vi "CRYCalc maximum.vi"(6 "Work in":u16, 7 "Step Setup VI No":i32, 8 "Statistic Run Number":i32, 11 "Data in":T1 {"Z data" items=["dB", "Lin"]; "X data" items=["dB", "Lin"]; "Y data" items=["dB", "Lin"]; "Z dB ref" format="%.1f"; "Z axis" items=["Log", "Lin"]; "X dB ref" format="%.1f"; "X axis" items=["Log", "Lin"]; "Y axis" items=["Log", "Lin"]; "Y dB ref" format="%.1f"; "Curve"."z" format="%.2f"; "Curve"."y" format="%.2f"; "Curve"."x" format="%.2f"}) -> (3 "Maximum Out":T1 {"Z data" items=["dB", "Lin"]; "X data" items=["dB", "Lin"]; "Y data" items=["dB", "Lin"]; "Z dB ref" format="%.1f"; "Z axis" items=["Log", "Lin"]; "X dB ref" format="%.1f"; "X axis" items=["Log", "Lin"]; "Y axis" items=["Log", "Lin"]; "Y dB ref" format="%.1f"; "Curve"."z" format="%.2f"; "Curve"."y" format="%.2f"; "Curve"."x" format="%.2f"})   [LabVIEW 2013]
uses:
  Typedef Control/CRYData Cluster Array.ctl
  Typedef Control/CRYData Cluster.ctl
  CRYStatistics Global.vi
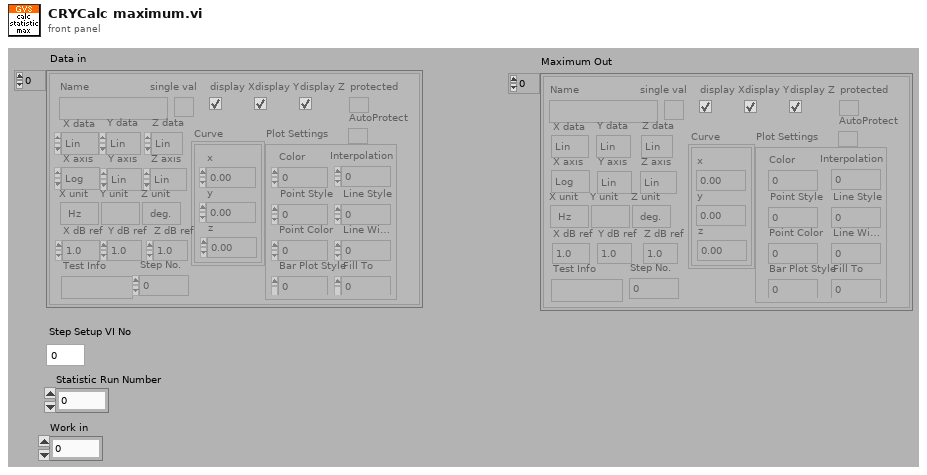
[diagram p1: front panel]
types:
  T1 = typedef "CRYData Cluster Array.ctl" = T2[]
  T2 = typedef "CRYData Cluster.ctl" = cluster{"Name":string, "Curve":cluster{"x":dbl, "y":dbl, "z":dbl}[], "X data":u16, "Y data":u16, "Z data":u16, "X axis":u16, "Y axis":u16, "Z axis":u16, "X unit":string, "Y unit":string, "Z unit":string, "X dB ref":dbl, "Y dB ref":dbl, "Z dB ref":dbl, "single val":bool, "protected":bool, "display X":bool, "display Y":bool, "display Z":bool, "Test Info":string, "Step No.":i32, "Plot Settings":cluster{"Color":u32, "Interpolation":u8, "Point Style":u8, "Line Style":u8, "Point Color":u32, "Line Width":u8, "Bar Plot Style":u8, "Fill To":i16}, "AutoProtect":bool}
  T3 = enum32{"English", "Chinese", "Korean", "Japanese", "Russian", "Chinese traditional"}
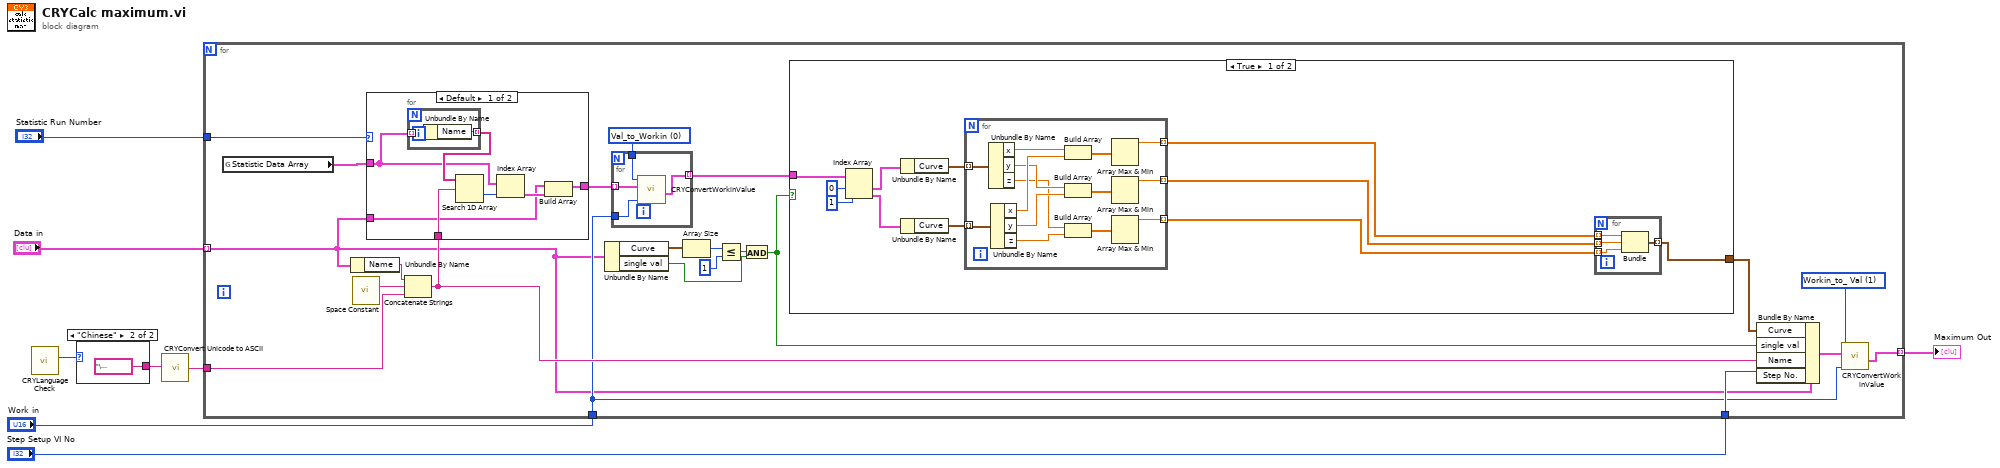
[diagram p0: block diagram]
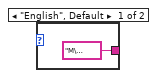
[diagram p2: hidden frame]
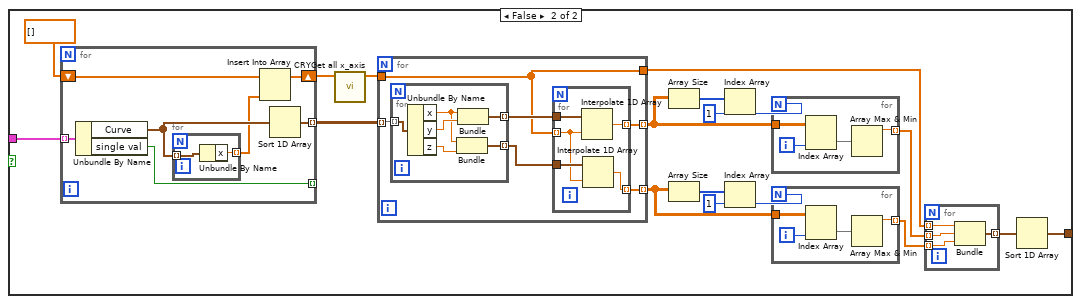
[diagram p3: hidden frame]
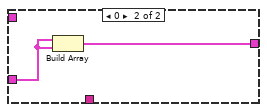
[diagram p4: hidden frame]
diagram:
  n1 = call "CRYLanguage Check.vi"() -> ("Language"=w4:T3)  [unwired: 10 in, 1 out]
  n2 = case shown="\"Chinese\"" w4 {
    tunnel: ["M\u0000a\u0000x\u0000" ("format string") "\u0000g'Y<P" ("format string")] -> w5
    frame "English", Default {
    }
    frame "Chinese" {
    }
  }
  n3 = call "CRYConvert Unicode to ASCII.vi"("Unicode"=w5) -> ("ASCII"=w3:string)  [unwired: 4 in]
  n4 = for {
    tunnel: "Data in" -> [w12] mode=indexing
    tunnel: [w21] -> w1 mode=indexing
    tunnel: "Step Setup VI No" -> [w30]
    tunnel: "Statistic Run Number" -> [w29]
    tunnel: w3 -> [w28]
    tunnel: "Work in" -> [w20]
    w18 = u16 1 items=["Val_to_Workin", "Workin_to_ Val"] ("Type")
    w19 = u16 0 items=["Val_to_Workin", "Workin_to_ Val"] ("Type")
    n5 = global read "CRYStatistics Global.vi" "Statistic Data Array"() -> (w25:T1)
    n6 = Unbundle By Name(w12) -> ("Name"=w26:string)
    n7 = call <vilib>:"Space Constant.vi"() -> ("String"=w27:string)
    n8 = Concatenate Strings(w26, w27, w28) -> (w31:string)
    n9 = case shown="Default" w29 {
      tunnel: w12 -> [w123 w132]
      tunnel: [w125 w131] -> w24
      tunnel: w31 -> [w128 _]
      tunnel: w25 -> [w122 _]
      frame Default {
        n10 = for {
          tunnel: w122 -> [w130] mode=indexing
          tunnel: [w129] -> w127 mode=indexing
          n11 = Unbundle By Name(w130) -> ("Name"=w129:string)
        }
        n12 = Search 1D Array(1D array=w127, element=w128) -> (index of element=w126:i32)  [unwired: 1 in]
        n13 = Index Array(array=w122, index=w126) -> (element=w124:T2)
        n14 = Build Array(w123, w124) -> (w125:T2[])
      }
      frame 0 {
        n15 = Build Array(w132, w132) -> (w131:T2[])
      }
    }
    n16 = Unbundle By Name(w12) -> ("Curve"=w13:cluster{"x":dbl, "y":dbl, "z":dbl}[], "single val"=w17:bool)
    n17 = for {
      tunnel: w24 -> [w121] mode=indexing
      tunnel: [w120] -> w23 mode=indexing
      tunnel: w19 -> [w119]
      tunnel: w20 -> [w118]
      n18 = call "CRYConvertWorkinValue.vi"("Work in"=w118, "In"=w121, "Type"=w119) -> ("Out"=w120:T2)  [unwired: 8 in]
    }
    n19 = Array Size(array=w13) -> (size(s)=w14:i32)
    n20 = Less Or Equal?(x=w14, y=1) -> (x <= y?=w16:bool)
    n21 = And(x=w16, y=w17) -> (x .and. y?=w11:bool)
    n22 = case shown="True" w11 {
      tunnel: [w33 w69] -> w32
      tunnel: w23 -> [w43 w62]
      frame True {
        n23 = Index Array(array=w43, index #1=0 ("index"), index #2=1 ("index")) -> (element #1=w40:T2, element #2=w39:T2)
        n24 = Unbundle By Name(w40) -> ("Curve"=w38:cluster{"x":dbl, "y":dbl, "z":dbl}[])
        n25 = Unbundle By Name(w39) -> ("Curve"=w37:cluster{"x":dbl, "y":dbl, "z":dbl}[])
        n26 = for {
          tunnel: w38 -> [w57] mode=indexing
          tunnel: w37 -> [w56] mode=indexing
          tunnel: [w46] -> w36 mode=indexing
          tunnel: [w45] -> w35 mode=indexing
          tunnel: [w44] -> w34 mode=indexing
          n27 = Unbundle By Name(w57) -> ("x"=w55:dbl, "y"=w53:dbl, "z"=w51:dbl)
          n28 = Unbundle By Name(w56) -> ("x"=w54:dbl, "y"=w52:dbl, "z"=w50:dbl)
          n29 = Build Array(w55, w54) -> (w49:dbl[])
          n30 = Build Array(w53, w52) -> (w48:dbl[])
          n31 = Build Array(w51, w50) -> (w47:dbl[])
          n32 = Array Max & Min(array=w49) -> (max value=w46:dbl)  [unwired: 3 out]
          n33 = Array Max & Min(array=w48) -> (max value=w45:dbl)  [unwired: 3 out]
          n34 = Array Max & Min(array=w47) -> (max value=w44:dbl)  [unwired: 3 out]
        }
        n35 = for {
          tunnel: [w61] -> w33 mode=indexing
          tunnel: w36 -> [w60] mode=indexing
          tunnel: w35 -> [w59] mode=indexing
          tunnel: w34 -> [w58] mode=indexing
          n36 = Bundle(w60, w59, w58) -> (w61:cluster{dbl, dbl, dbl})  [unwired: 1 out]
        }
      }
      frame False {
        n37 = for {
          tunnel: [w92] -> w76 mode=indexing
          tunnel: w62 -> [w93] mode=indexing
          shift-right: [w96] -> w68
          shift-left: dbl[] [] ("x_Array") -> [w95]
          tunnel: [w94] -> _ mode=indexing
          n38 = Unbundle By Name(w93) -> ("Curve"=w98:cluster{"x":dbl, "y":dbl, "z":dbl}[], "single val"=w94:bool)
          n39 = for {
            tunnel: w98 -> [w99] mode=indexing
            tunnel: [w100] -> w97 mode=indexing
            n40 = Unbundle By Name(w99) -> ("x"=w100:dbl)
          }
          n41 = Insert Into Array(array=w95, new element=w97) -> (w96:dbl[])  [unwired: 1 in]
          n42 = Sort 1D Array(array=w98) -> (sorted array=w92:cluster{"x":dbl, "y":dbl, "z":dbl}[])
        }
        n43 = call "CRYGet all x_axis.vi"("x_Array in"=w68) -> ("X_axis out"=w75:dbl[])  [unwired: 1 in, 9 out]
        n44 = for {
          tunnel: w76 -> [w102] mode=indexing
          tunnel: [w106] -> w78 mode=indexing
          tunnel: w75 -> [w101]
          tunnel: [w101] -> w79
          tunnel: [w103] -> w64 mode=indexing
          n45 = for {
            tunnel: [w111] -> w105 mode=indexing
            tunnel: w102 -> [w110] mode=indexing
            tunnel: [w107] -> w104 mode=indexing
            n46 = Unbundle By Name(w110) -> ("x"=w108:dbl, "y"=w112:dbl, "z"=w109:dbl)
            n47 = Bundle("x"=w108, "z"=w109) -> (w107:cluster{"x":dbl, "z":dbl})  [unwired: 1 out]
            n48 = Bundle("x"=w108, "y"=w112) -> (w111:cluster{"x":dbl, "y":dbl})  [unwired: 1 out]
          }
          n49 = for {
            tunnel: [w117] -> w106 mode=indexing
            tunnel: w105 -> [w116]
            tunnel: w101 -> [w114] mode=indexing
            tunnel: w104 -> [w115]
            tunnel: [w113] -> w103 mode=indexing
            n50 = Interpolate 1D Array(1:w114, 2:w116) -> (0:w117:dbl)
            n51 = Interpolate 1D Array(1:w114, 2:w115) -> (0:w113:dbl)
          }
        }
        n52 = Array Size(array=w78) -> (size(s)=w74:i32[])
        n53 = Array Size(array=w64) -> (size(s)=w65:i32[])
        n54 = Index Array(array=w74, index=1) -> (element=w73:i32)
        n55 = Index Array(array=w65, index=1) -> (element=w66:i32)
        n56 = for {
          N: w73 -> [_]
          tunnel: w78 -> [w91]
          tunnel: [w89] -> w71 mode=indexing
          i -> [w88]
          n57 = Index Array(array=w91, index (col)=w88) -> (element=w90:dbl[])  [unwired: 1 in]
          n58 = Array Max & Min(array=w90) -> (max value=w89:dbl)  [unwired: 3 out]
        }
        n59 = for {
          N: w66 -> [_]
          tunnel: w64 -> [w83]
          tunnel: [w81] -> w63 mode=indexing
          i -> [w80]
          n60 = Index Array(array=w83, index (col)=w80) -> (element=w82:dbl[])  [unwired: 1 in]
          n61 = Array Max & Min(array=w82) -> (max value=w81:dbl)  [unwired: 3 out]
        }
        n62 = for {
          tunnel: w71 -> [w86] mode=indexing
          tunnel: [w87] -> w70 mode=indexing
          tunnel: w79 -> [w85] mode=indexing
          tunnel: w63 -> [w84] mode=indexing
          n63 = Bundle("x"=w85, w86, w84) -> (w87:cluster{"x":dbl, dbl, dbl})  [unwired: 1 out]
        }
        n64 = Sort 1D Array(array=w70) -> (sorted array=w69:cluster{"x":dbl, dbl, dbl}[])
      }
    }
    n65 = Bundle By Name(cluster=w12, "Curve"=w32, "single val"=w11, "Name"=w31, "Step No."=w30) -> (w22:T2)
    n66 = call "CRYConvertWorkinValue.vi"("Work in"=w20, "In"=w22, "Type"=w18) -> ("Out"=w21:T2)  [unwired: 8 in]
  }
  "Maximum Out" <- w1
